vi "speed&col syncroun 2.vi"(0 "speed array in":dbl[](array[numeric]), 1 "speed":dbl, 2 "width":dbl, 3 "start":bool, 4 "instant capture":bool, 5 "acceptable width":dbl, 6 "plt count":bool, 7 "error in (no error)":errorcluster) -> (14 "total movement":dbl, 15 "Elapsed Time (s)":dbl, 16 "speed array out":dbl[](array[numeric]), 17 "speed triger":bool, 18 "plt count accept":bool, 19 "error out":errorcluster)   [LabVIEW 2019]
uses:
  <vilib>/measure/mamon.llb/Trigger Detection for 1 Channel.vi
  <vilib>/measure/NI_MAPro.lvlib
panel:
  out "previous movment":dbl
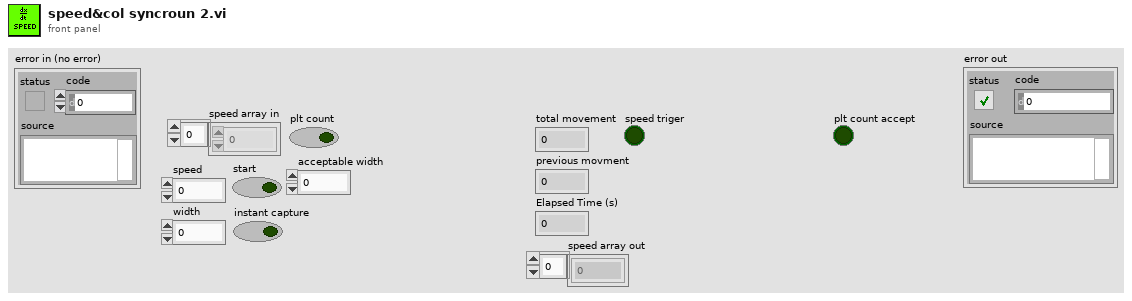
[diagram p1: front panel]
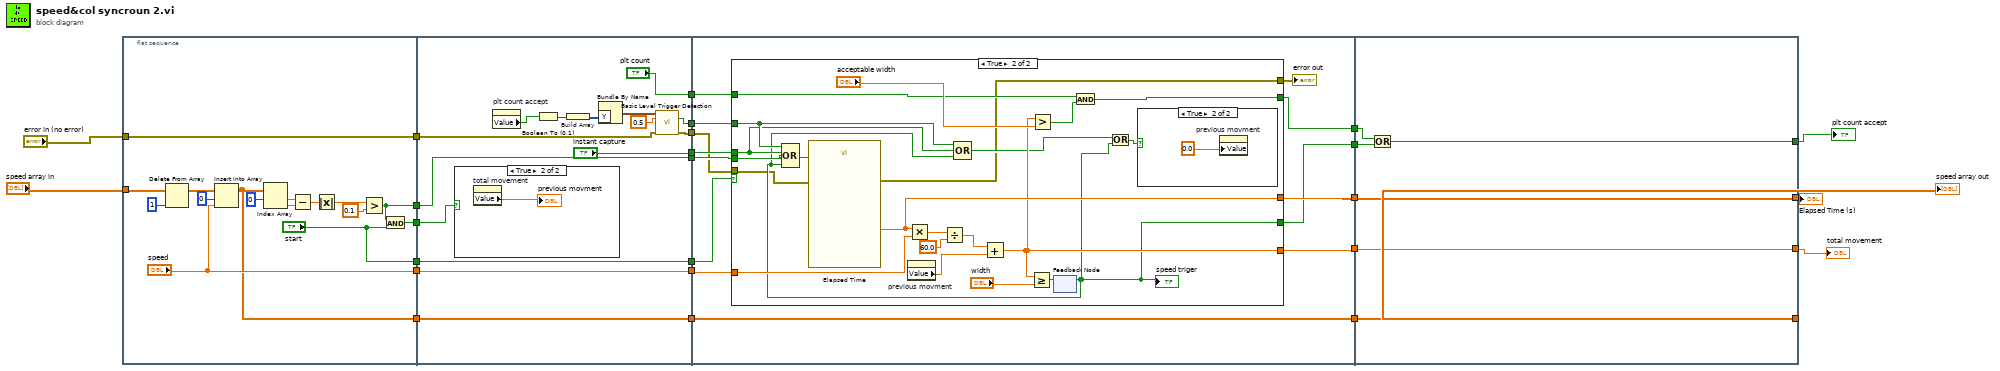
[diagram p0: block diagram]
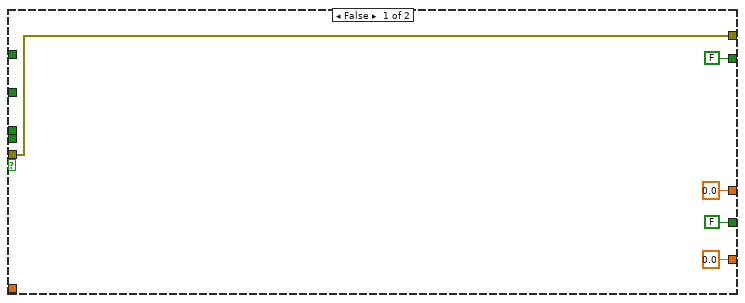
[diagram p3: hidden frame]
diagram:
  n1 = flat-sequence {
    tunnel: "speed array in" -> [w40]
    tunnel: [w29] -> w23
    tunnel: ["speed"] -> w22
    tunnel: [w30] -> w21
    tunnel: [w28] -> w20
    tunnel: ["start"] -> w19
    tunnel: [w27] -> w3
    tunnel: "error in (no error)" -> [w27]
    tunnel: w23 -> [w56]
    tunnel: [w56] -> w18
    tunnel: [w55] -> w17
    tunnel: w22 -> [w55]
    tunnel: [w54] -> w16
    tunnel: w21 -> [w54]
    tunnel: w20 -> [w53]
    tunnel: [w52] -> w15
    tunnel: w19 -> [w52]
    tunnel: ["instant capture"] -> w14
    tunnel: ["plt count"] -> w13
    tunnel: [w45] -> w12
    tunnel: w3 -> [w44]
    tunnel: [w43] -> w1
    tunnel: w18 -> [w70]
    tunnel: w17 -> [w69]
    tunnel: w16 -> [w67]
    tunnel: w15 -> [w65]
    tunnel: w14 -> [w64]
    tunnel: w13 -> [w63]
    tunnel: w12 -> [w62]
    tunnel: [w68] -> w11
    tunnel: [w66] -> w10
    tunnel: [w67] -> w9
    tunnel: [w61] -> w8
    tunnel: [w60] -> w7
    tunnel: w1 -> [w59]
    tunnel: [w102] -> w25
    tunnel: [w103] -> w6
    tunnel: [w104] -> w5
    tunnel: w11 -> [w104]
    tunnel: w10 -> [w103]
    tunnel: w9 -> [w102]
    tunnel: w8 -> [w101]
    tunnel: w7 -> [w100]
    tunnel: [w99] -> w4
    frame #0 {
      n2 = Delete From Array(array=w40, index=1) -> (array with subset deleted=w34:dbl[])  [unwired: 1 in, 1 out]
      n3 = Insert Into Array(array=w34, index=0, new element="speed") -> (w30:dbl[])
      n4 = Index Array(array=w30, index #1=0 ("index")) -> (element #1=w33:dbl, element #2=w32:dbl)  [unwired: 1 in]
      n5 = Subtract(x=w33, y=w32) -> (x-y=w38:dbl)
      n6 = Absolute Value(x=w38) -> (abs(x)=w39:dbl)
      n7 = Greater?(x=w39, y=0.1) -> (0:w29:bool)
      n8 = And(x=w29, y="start") -> (x .and. y?=w28:bool)
    }
    frame #1 {
      n9 = case shown="True" w53 {
        frame False {
        }
        frame True {
          n10 = property on="total movement" class="DigNum (strict)"() -> ("Value"=→"previous movment":dbl)  [unwired: 2 in, 2 out]
        }
      }
      n11 = property on="plt count accept" class="Bool (strict)"() -> ("Value"=w46:bool)  [unwired: 2 in, 2 out]
      n12 = Boolean To (0,1)(Boolean=w46) -> (0, 1=w48:i16)
      n13 = Build Array(w48) -> (w49:i16[])
      n14 = Bundle By Name("Y"=w49) -> (w50:waveform(i16))  [unwired: 1 in]
      n15 = call-poly <vilib>:"Basic Level Trigger Detection.vi"("signal in"=w50, "level"=0.5, "error in (no error)"=w44) -> ("trigger detected?"=w45:bool, "error out"=w43:errorcluster)  [unwired: 10 in, 1 out]
    }
    frame #2 {
      n16 = case shown="True" w65 {
        tunnel: w70 -> [_ w97]
        tunnel: w69 -> [_ w96]
        tunnel: [0.0 w86] -> w68
        tunnel: [0.0 ("Elapsed Time (s)") w89] -> w66
        tunnel: w64 -> [_ w80]
        tunnel: w63 -> [_ w82]
        tunnel: [FALSE w85] -> w61
        tunnel: w62 -> [_ w81]
        tunnel: [FALSE w79] -> w60
        tunnel: w59 -> [w71 w77]
        tunnel: [w71 w76] -> w58
        frame False {
        }
        frame True {
          n17 = property on="previous movment" class="DigNum (strict)"() -> ("Value"=w90:dbl)  [unwired: 2 in, 2 out]
          n18 = feedback #1() -> (w79:bool)  [unwired: 1 in]
          "speed triger" <- w79
          n19 = Compound Arithmetic op=OR(w81, w80, w97, w79) -> (w83:bool)
          n20 = call "Elapsed Time"("Reset"=w83, "error in (no error)"=w77) -> ("Elapsed Time (s)"=w89:dbl, "error out"=w76:errorcluster)  [unwired: 10 in, 6 out]
          n21 = Multiply(x=w89, y=w96) -> (x*y=w95:dbl)
          n22 = Divide(x=w95, y=60.0) -> (x/y=w93:dbl)
          n23 = Compound Arithmetic op=OR(w81, w80, w79) -> (w78:bool)
          n24 = Add(x=w93, y=w90) -> (x+y=w86:dbl)
          n25 = Greater Or Equal?(x=w86, y="width") -> (x >= y?=w91:bool)
          n26 = Greater?(x=w86, y="acceptable width") -> (0:w87:bool)
          n27 = feedback-in #1(w91) -> ()
          n28 = And(x=w82, y=w87) -> (x .and. y?=w85:bool)
          n29 = Or(x=w78, y=w79) -> (x .or. y?=w84:bool)
          n30 = case shown="True" w84 {
            frame False {
            }
            frame True {
              n31 = property on="previous movment" class="DigNum (strict)"("Value"=0.0 ("previous movment")) -> ()  [unwired: 2 in, 2 out]
            }
          }
        }
      }
      "error out" <- w58
    }
    frame #3 {
      n32 = Or(x=w101, y=w100) -> (x .or. y?=w99:bool)
    }
  }
  "speed array out" <- w25
  "Elapsed Time (s)" <- w6
  "total movement" <- w5
  "plt count accept" <- w4
